vi "Store Block Measurements.vi"(8 "error in (no error)":errorcluster, 10 "Number of readings (10)":i32=10, 11 "VISA resource name":refnum<visa-resource-name>) -> (0 "error out":errorcluster, 3 "VISA resource name out":refnum<visa-resource-name>)   [LabVIEW 2011, in "Fluke 8508.lvlib"]
doc: "This VI stores the specified number of readings into the internal buffer of the instrument.\n\n<B>NOTES</B>\n(1) When the instrument is initialized, power cycled or when this VI is run, all previously stored data will be removed / overwritten.\n(2) If the trigger mode is set to \"external\" in the Configure Trigger VI, the instrument will wait for n number of triggers equivalent to the number of readings specified. Therefore, in the external trigger mode it is necessary to send all the triggers before reading the data buffer on the instrument. (A trigger can be sent using the \"Send Software Trigger\" VI, and the stored data can be read using the \"Read Block Measurements\" VI)"
uses:
  Fluke 8508.lvlib
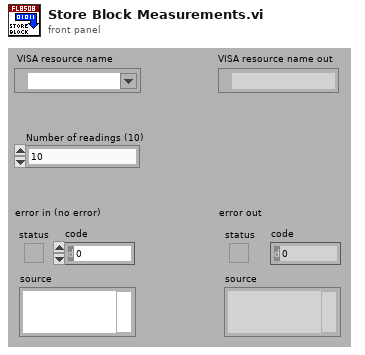
[diagram p1: front panel]
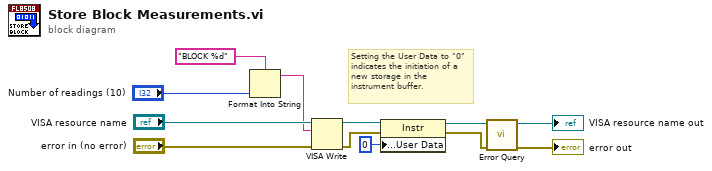
[diagram p0: block diagram]
diagram:
  # "Setting the User Data to \"0\" indicates the initiation of a new storage in the instrument buffer."
  n1 = Format Into String(format string="BLOCK %d", "Number of readings (10)") -> (resulting string=w9:string)  [unwired: 2 in, 1 out]
  n2 = VISA Write(VISA resource name="VISA resource name", write buffer=w9, error in (no error)="error in (no error)") -> (VISA resource name out=w8:refnum<visa-resource-name>, error out=w7:errorcluster)  [unwired: 1 out]
  n3 = property class="Instr"(reference=w8, error in=w7, "General Settings:User Data"=u32 0) -> (reference out=w3:refnum<visa-resource-name>, error out=w2:errorcluster)
  n4 = call "Error Query.vi"("error in (no error)"=w2, "VISA resource name"=w3) -> ("error out"=→"error out":errorcluster, "VISA resource name out"=→"VISA resource name out":refnum<visa-resource-name>)  [unwired: 6 in, 2 out]
